vi "main_error_report.vi"(8 "error in":errorcluster, 11 "TabCtl Refnum":refnum<vi>) -> (3 "message":string)   [LabVIEW 2010]
uses:
  <vilib>/Utility/error.llb/DialogType.ctl
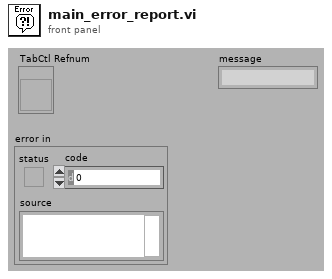
[diagram p1: front panel]
types:
  T1 = typedef "DialogType.ctl" = u16
  T2 = enum32{"scanHead", "imagingMode", "daq", "imageAssembler", "dataCollection", "analysis", "experimentController", "stimulator", "stage", "instrument", "errorLog"}
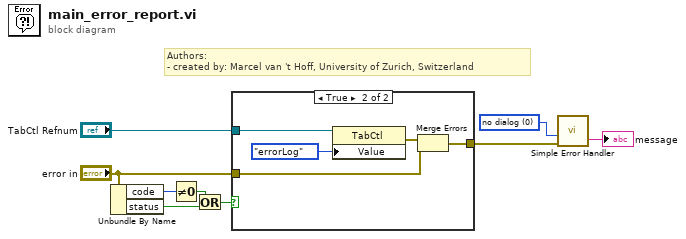
[diagram p0: block diagram]
diagram:
  w8 = T1 0 items=["no dialog", "OK message", "continue or stop message", "OK message + warnings", "continue/stop + warnings"] ("type of dialog (OK msg:1)")
  # "Authors: \n- created by: Marcel van 't Hoff, University of Zurich, Switzerland"
  n1 = Unbundle By Name("error in") -> ("code"=w4:i32, "status"=w3:bool)
  n2 = Not Equal To 0?(x=w4) -> (x != 0?=w2:bool)
  n3 = Or(x=w2, y=w3) -> (x .or. y?=w1:bool)
  n4 = case shown="True" w1 {
    tunnel: [w10 w12] -> w7
    tunnel: "TabCtl Refnum" -> [_ w14]
    tunnel: "error in" -> [w10 w11]
    frame False {
    }
    frame True {
      n5 = property class="TabCtl"(reference=w14, "Value"=T2."errorLog" ("settings tab")) -> (error out=w15:errorcluster)  [unwired: 1 in, 1 out]
      n6 = Merge Errors(w15, w11) -> (w12:errorcluster)
    }
  }
  n7 = call <vilib>:"Simple Error Handler.vi"("type of dialog (OK msg:1)"=w8, "error in (no error)"=w7) -> ("message"=→"message":string)  [unwired: 7 out]
